vi "Array to File.vi"(8 "error in":errorcluster, 10 "array in":T1[](array[typedef]) {"Creation Date" format="%<%x>T"; "Last Updated" format="%<%x>T"}, 11 "file path in":path) -> (0 "error out":errorcluster, 3 "file path out":path)   [LabVIEW 2018]
uses:
  Type Defs/SR Cluster.ctl
  Type Defs/SR Status.ctl
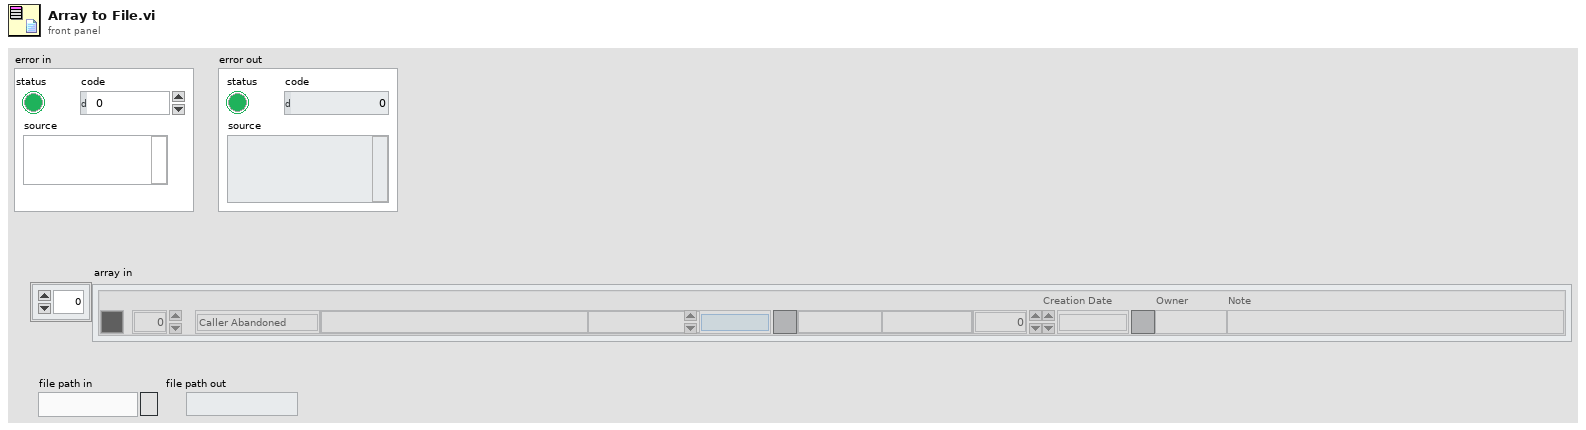
[diagram p1: front panel]
types:
  T1 = typedef "SR Cluster.ctl" = cluster{"Color":u32, "SR Number":i32, "SR Status":T2, "Name":string, "Summary":string, "Last Updated":timestamp, "SR Type":string, "Service Level":string, "Days Open":dbl, "Creation Date":timestamp, "Owner":string, "Note":string}
  T2 = typedef "SR Status.ctl" = enum16{"Caller Abandoned", "Created in Error", "Expired", "Forum Resolved AE", "Forum Resolved Customer", "IN WORK", "IN WORK Collab with AES", "IN WORK Collab with PSE", "IN WORK Collab with SE", "IN WORK Customer Added Note", "IN WORK Escalation", "IN WORK Wait on Customer", "Open", "Potentially Resolved", "Presumed Resolved", "RMA Approved for Return", "RMA Closed", "RMA Closed - DOA", "RMA In Progress", "RMA Open", "RMA Waiting on Customer", "Resolved", "Passed Off"}
  T3 = enum16{"open", "replace", "create", "open or create", "replace or create", "replace or create with confirmation"}
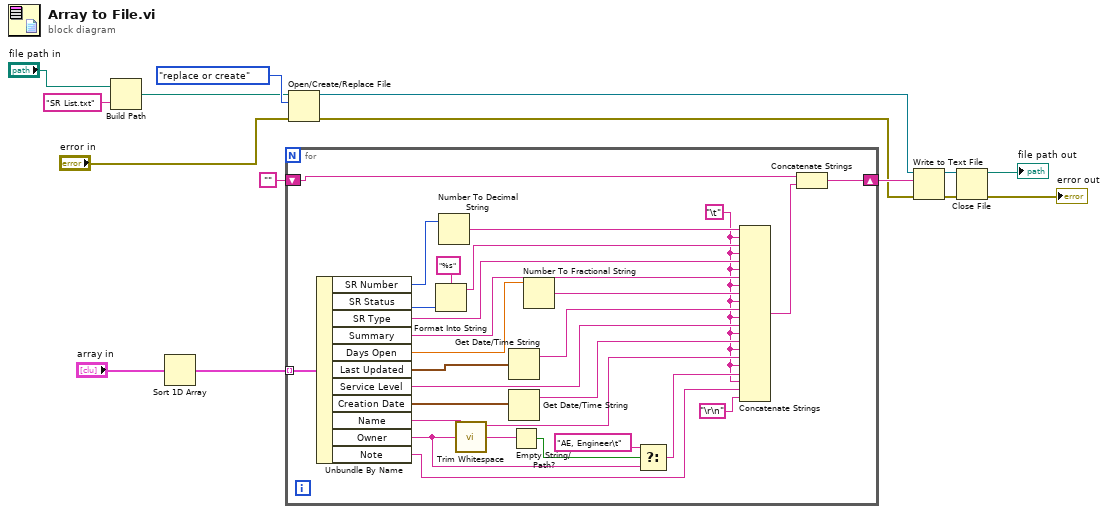
[diagram p0: block diagram]
diagram:
  n1 = Build Path(base path="file path in", name or relative path="SR List.txt") -> (appended path=w1:path)
  n2 = Sort 1D Array(array="array in") -> (sorted array=w4:T1[])
  n3 = for {
    shift-right: [w42] -> w13
    shift-left: "" -> [w41]
    tunnel: w4 -> [w27] mode=indexing
    w18 = "\t"
    n4 = Unbundle By Name(w27) -> ("SR Number"=w39:i32, "SR Status"=w30:T2, "SR Type"=w37:string, "Summary"=w31:string, "Days Open"=w36:dbl, "Last Updated"=w32:timestamp, "Service Level"=w33:string, "Creation Date"=w26:timestamp, "Name"=w24:string, "Owner"=w21:string, "Note"=w17:string)
    n5 = Format Into String(format string="%s", w30) -> (resulting string=w28:string)  [unwired: 2 in, 1 out]
    n6 = Number To Decimal String(number=w39) -> (decimal integer string=w38:string)  [unwired: 1 in]
    n7 = call <vilib>:"Trim Whitespace.vi"("string"=w21) -> ("trimmed string"=w23:string)  [unwired: 1 in]
    n8 = Get Date/Time String(seconds (now)=w32) -> (date string=w34:string)  [unwired: 2 in, 1 out]
    n9 = Get Date/Time String(seconds (now)=w26) -> (date string=w25:string)  [unwired: 2 in, 1 out]
    n10 = Empty String/Path?(string/path=w23) -> (empty?=w22:bool)
    n11 = Number To Fractional String(number=w36) -> (F-format string=w35:string)  [unwired: 3 in]
    n12 = Select(t="AE, Engineer\t", s=w22, f=w21) -> (s? t:f=w19:string)
    n13 = Concatenate Strings(w38, w18, w28, w18, w37, w18, w31, w18, w35, w18, w34, w18, w33, w18, w25, w18, w24, w18, w19, w18, w17, "\r\n") -> (w40:string)
    n14 = Concatenate Strings(w41, w40) -> (w42:string)
  }
  n15 = Open/Create/Replace File(file path (use dialog)=w1, error in="error in", operation (0:open)=T3."replace or create") -> (refnum out=w11:refnum<file>, error out=w12:errorcluster)  [unwired: 3 in, 1 out]
  n16 = Write to Text File(file (use dialog)=w11, text=w13, error in=w12) -> (refnum out=w9:refnum<file>, error out=w10:errorcluster)  [unwired: 1 in, 1 out]
  n17 = Close File(refnum=w9, error in=w10) -> (path=→"file path out":path, error out=→"error out":errorcluster)
